vi "Read SelectedPropertyHierarchy.vi"(8 "error in (no error)":errorcluster, 11 "TektronixDPO in":refnum<class "TektronixDPO.lvclass">) -> (0 "error out":errorcluster, 2 "SelectedPropertyHierarchy":string[](array[string]), 3 "TektronixDPO out":refnum<class "TektronixDPO.lvclass">)   [LabVIEW 2013, in "TektronixDPO.lvclass"]
uses:
  TektronixDPO.lvclass
  TektronixDPO.lvclass/TektronixDPO.ctl
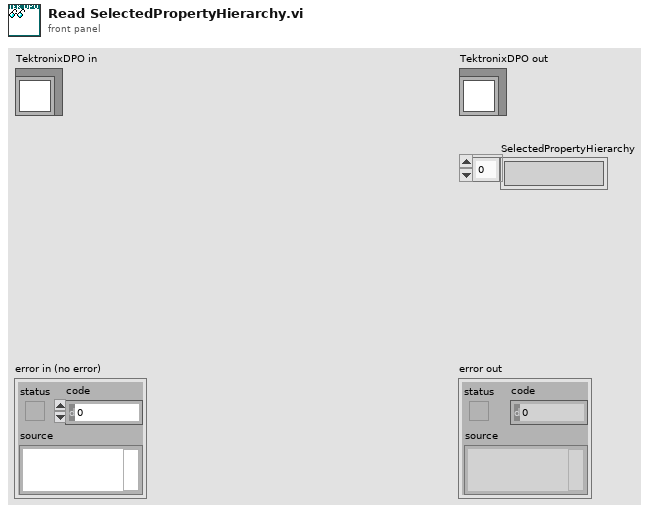
[diagram p1: front panel]
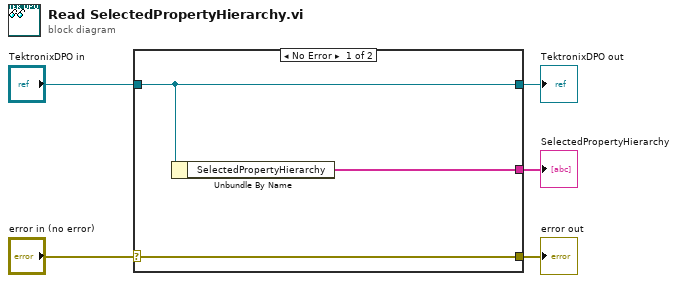
[diagram p0: block diagram]
diagram:
  n1 = case shown="No Error" "error in (no error)" {
    selector: "error in (no error)" -> [w8 w9]
    tunnel: [w8 w9] -> w4
    tunnel: [w7 w10] -> w2
    tunnel: "TektronixDPO in" -> [w7 w10]
    tunnel: [w6 _] -> w1
    frame No Error {
      n2 = Unbundle By Name(w7) -> ("SelectedPropertyHierarchy"=w6:string[])
    }
    frame Error {
    }
  }
  "error out" <- w4
  "TektronixDPO out" <- w2
  "SelectedPropertyHierarchy" <- w1
